vi "Scanner.vi"(7 "Inc:(um)":dbl, 8 "error in (no error)":errorcluster caption="entrée d'erreur (pas d'erreur)", 11 "UI SA en entrée":refnum<class "UI SmarAct.lvclass">) -> (0 "error out":errorcluster caption="sortie d'erreur", 2 "Nbre de scans":i32, 3 "UI SA en sortie":refnum<class "UI SmarAct.lvclass">)   [LabVIEW 2024, in "UI SmarAct.lvclass"]
uses:
  UI SmarAct.lvclass
  Spectro Acquisition/rqp_Init One Acquisition.ctl
  UI SmarAct.lvclass/UI SmarAct.ctl
  <vilib>/Analysis/1siggen.llb/Ramp Pattern by Samples.vi
  <vilib>/Utility/error.llb/Error Cluster From Error Code.vi
  <vilib>/ErrorRing/Error Ring.xnode
  Spectro Acquisition/Spectro Acquisition.lvclass
  <vilib>/Analysis/NI_AALBase.lvlib
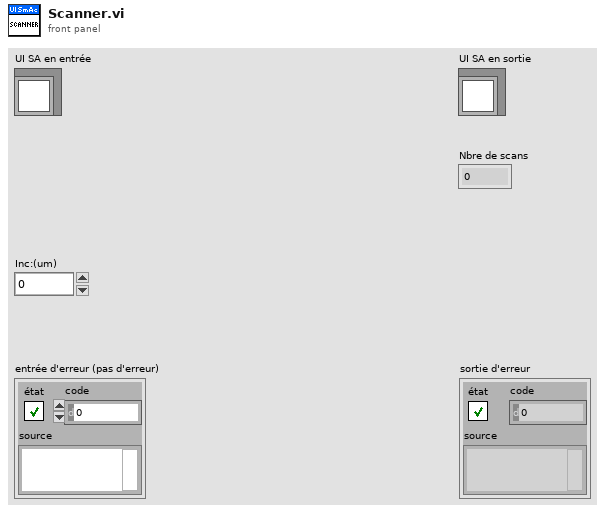
[diagram p1: front panel]
types:
  T1 = typedef "Spectro Acquisition.lvclass/rqp_Init One Acquisition.ctl" = cluster{"Init Incrément":i32}
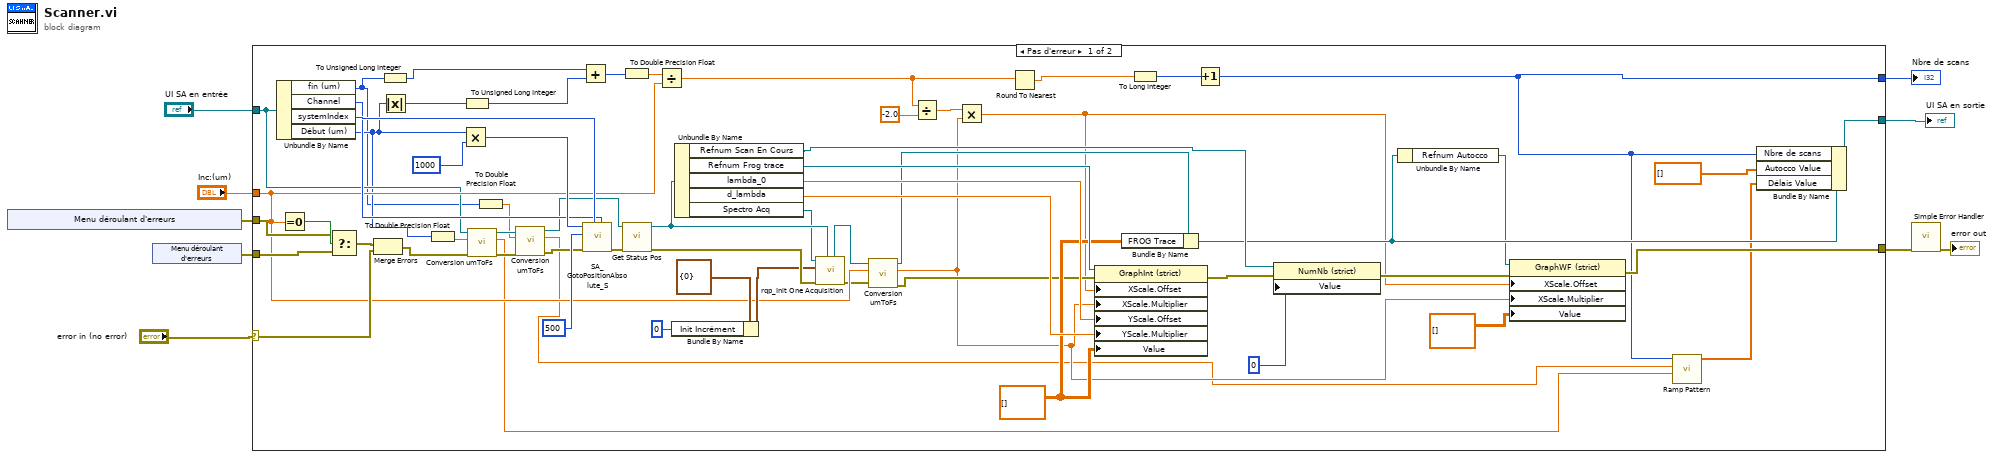
[diagram p0: block diagram]
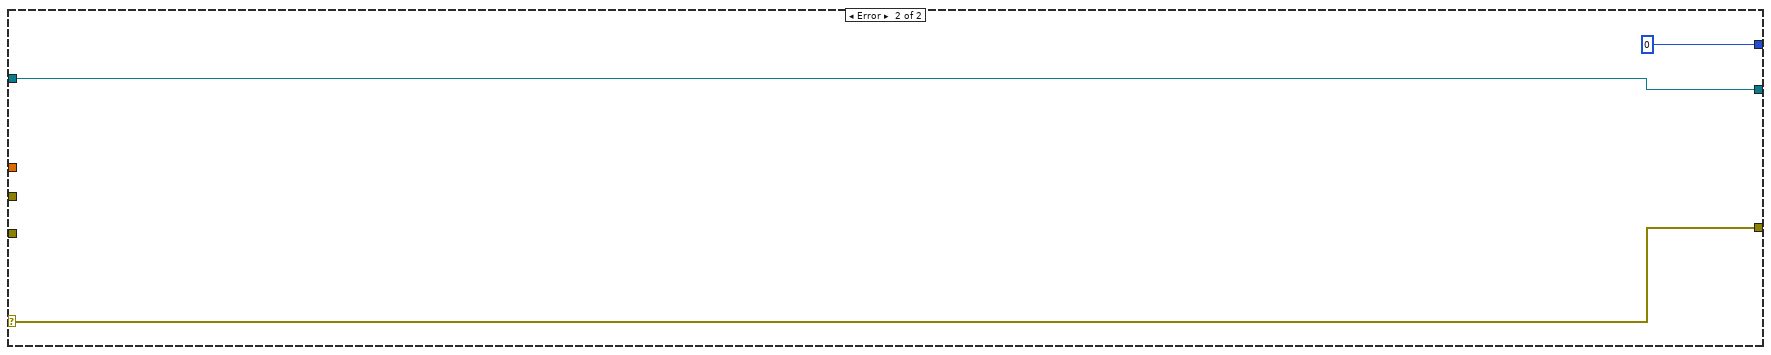
[diagram p2: hidden frame]
diagram:
  n1 = xnode "Menu déroulant d'erreurs"() -> ("sortie d'erreur"=w5:errorcluster)
  n2 = xnode "Menu déroulant d'erreurs"() -> ("sortie d'erreur"=w4:errorcluster)
  n3 = case shown="Pas d'erreur" "error in (no error)" {
    selector: "error in (no error)" -> [w67 w74]
    tunnel: [w32 w74] -> w2
    tunnel: [w34 w73] -> w7
    tunnel: "UI SA en entrée" -> [w21 w73]
    tunnel: "Inc:(um)" -> [w47 _]
    tunnel: w5 -> [w64 _]
    tunnel: w4 -> [w63 _]
    tunnel: [w15 0] -> w3
    frame No Error {
      w44 = dbl[][] [] ("FROG Trace")
      n4 = Unbundle By Name(w21) -> ("fin (um)"=w17:i32, "Channel"=w58:u32, "systemIndex"=w59:u32, "Début (um)"=w19:i32)
      n5 = Equal To 0?(x=w47) -> (x = 0?=w66:bool)
      n6 = Select(t=w64, s=w66, f=w63) -> (s? t:f=w65:errorcluster)
      n7 = Merge Errors(w65, w67) -> (w22:errorcluster)
      n8 = To Unsigned Long Integer(number=w17) -> (unsigned 32bit integer=w38:u32)
      n9 = Absolute Value(x=w19) -> (abs(x)=w71:i32)
      n10 = To Double Precision Float(number=w19) -> (double precision float=w18:dbl)
      n11 = Multiply(x=w19, y=1000 ("holdTime")) -> (x*y=w60:i32)
      n12 = To Unsigned Long Integer(number=w71) -> (unsigned 32bit integer=w39:u32)
      n13 = call "Conversion umToFs.vi"("error in (no error)"=w22, "um"=w18, "UI SA en entrée"=w21) -> ("error out"=w25:errorcluster, "Fs"=w14:ext, "UI SA en sortie"=w24:refnum<class "UI SmarAct.lvclass">)  [unwired: 6 in]
      n14 = To Double Precision Float(number=w17) -> (double precision float=w16:dbl)
      n15 = call "Conversion umToFs.vi"("error in (no error)"=w25, "um"=w16, "UI SA en entrée"=w24) -> ("error out"=w23:errorcluster, "Fs"=w13:ext, "UI SA en sortie"=w20:refnum<class "UI SmarAct.lvclass">)  [unwired: 6 in]
      n16 = Add(x=w38, y=w39) -> (x+y=w70:u32)
      n17 = call <vilib>:"SA_GotoPositionAbsolute_S.vi"("channelIndex"=w58, "systemIndex"=w59, "error in (no error)"=w23, "holdTime"=u32 500, "position"=w60) -> ("error out"=w57:errorcluster)  [unwired: 6 in]
      n18 = To Double Precision Float(number=w70) -> (double precision float=w69:dbl)
      n19 = call "Get Status Pos.vi"("error in (no error)"=w57, "UI SA en entrée"=w20) -> ("error out"=w56:errorcluster, "UI SA en sortie"=w55:refnum<class "UI SmarAct.lvclass">)  [unwired: 8 in]
      n20 = Divide(x=w69, y=w47) -> (x/y=w68:dbl)
      n21 = Bundle By Name(cluster=T1 {"Init Incrément"=0} ("Data in"), "Init Incrément"=0) -> (w52:T1)
      n22 = Unbundle By Name(w55) -> ("Refnum Scan En Cours"=w37:refnum<vi>, "Refnum Frog trace"=w50:refnum<vi>, "lambda_0"=w46:dbl, "d_lambda"=w45:dbl, "Spectro Acq"=w54:refnum<class "Spectro Acquisition.lvclass">)
      n23 = call "rqp_Init One Acquisition.vi"("Caller in"=w55, "error in"=w56, "Data in"=w52, "Spectro Acquisition in"=w54) -> ("error out"=w41:errorcluster, "dup Caller out"=w43:refnum<class "UI SmarAct.lvclass">)  [unwired: 5 in, 1 out]
      n24 = call "Conversion umToFs.vi"("error in (no error)"=w41, "um"=w47, "UI SA en entrée"=w43) -> ("error out"=w40:errorcluster, "Fs"=w27:ext, "UI SA en sortie"=w42:refnum<class "UI SmarAct.lvclass">)  [unwired: 6 in]
      n25 = Divide(x=w68, y=-2.0) -> (x/y=w48:dbl)
      n26 = Multiply(x=w48, y=w27) -> (x*y=w28:ext)
      n27 = Round To Nearest(number=w68) -> (nearest integer value=w10:dbl)
      n28 = property class="GraphInt (strict)"(reference=w50, error in=w40, "XScale.Offset"=w28, "XScale.Multiplier"=w27, "YScale.Offset"=w46, "YScale.Multiplier"=w45, "Value"=w44) -> (error out=w35:errorcluster)  [unwired: 1 out]
      n29 = Bundle By Name(cluster=w42, "FROG Trace"=w44) -> (w30:refnum<class "UI SmarAct.lvclass">)
      n30 = To Long Integer(number=w10) -> (32bit integer=w33:i32)
      n31 = Increment(x=w33) -> (x+1=w15:i32)
      n32 = property class="NumNb (strict)"(reference=w37, error in=w35, "Value"=0 ("Valeur")) -> (error out=w31:errorcluster)  [unwired: 1 out]
      n33 = Unbundle By Name(w30) -> ("Refnum Autocco"=w29:refnum<vi>)
      n34 = property class="GraphWF (strict)"(reference=w29, error in=w31, "XScale.Offset"=w28, "XScale.Multiplier"=w27, "Value"=dbl[][] [] ("Valeur")) -> (error out=w32:errorcluster)  [unwired: 1 out]
      n35 = call-poly <vilib>:"Ramp Pattern.vi"("start"=w14, "end"=w13, "samples"=w15) -> ("Ramp Pattern"=w12:dbl[])  [unwired: 7 in, 1 out]
      n36 = Bundle By Name(cluster=w30, "Nbre de scans"=w15, "Autocco Value"=dbl[] [] ("Valeur"), "Délais Value"=w12) -> (w34:refnum<class "UI SmarAct.lvclass">)
    }
    frame Error {
    }
  }
  "UI SA en sortie" <- w7
  "Nbre de scans" <- w3
  n37 = call <vilib>:"Simple Error Handler.vi"("error in (no error)"=w2) -> ("error out"=→"error out":errorcluster)  [unwired: 4 in, 4 out]
